vi "main(debug2_chagne_gen3_format).vi"() -> ()   [LabVIEW 2015]
panel:
  out "삭제된 부분":string[][](array[string])
  out "Filtered Sensor":u32[][](array[numeric])
  out "No Filter Sensor":u32[][](array[numeric])
  out "Time":string[](array[string])
  out "배열":string[](array[string])
  in  "패턴(*.txt)":string="*.txt"
  out "파일 이름":string[](array[string])
  in  "경로":path
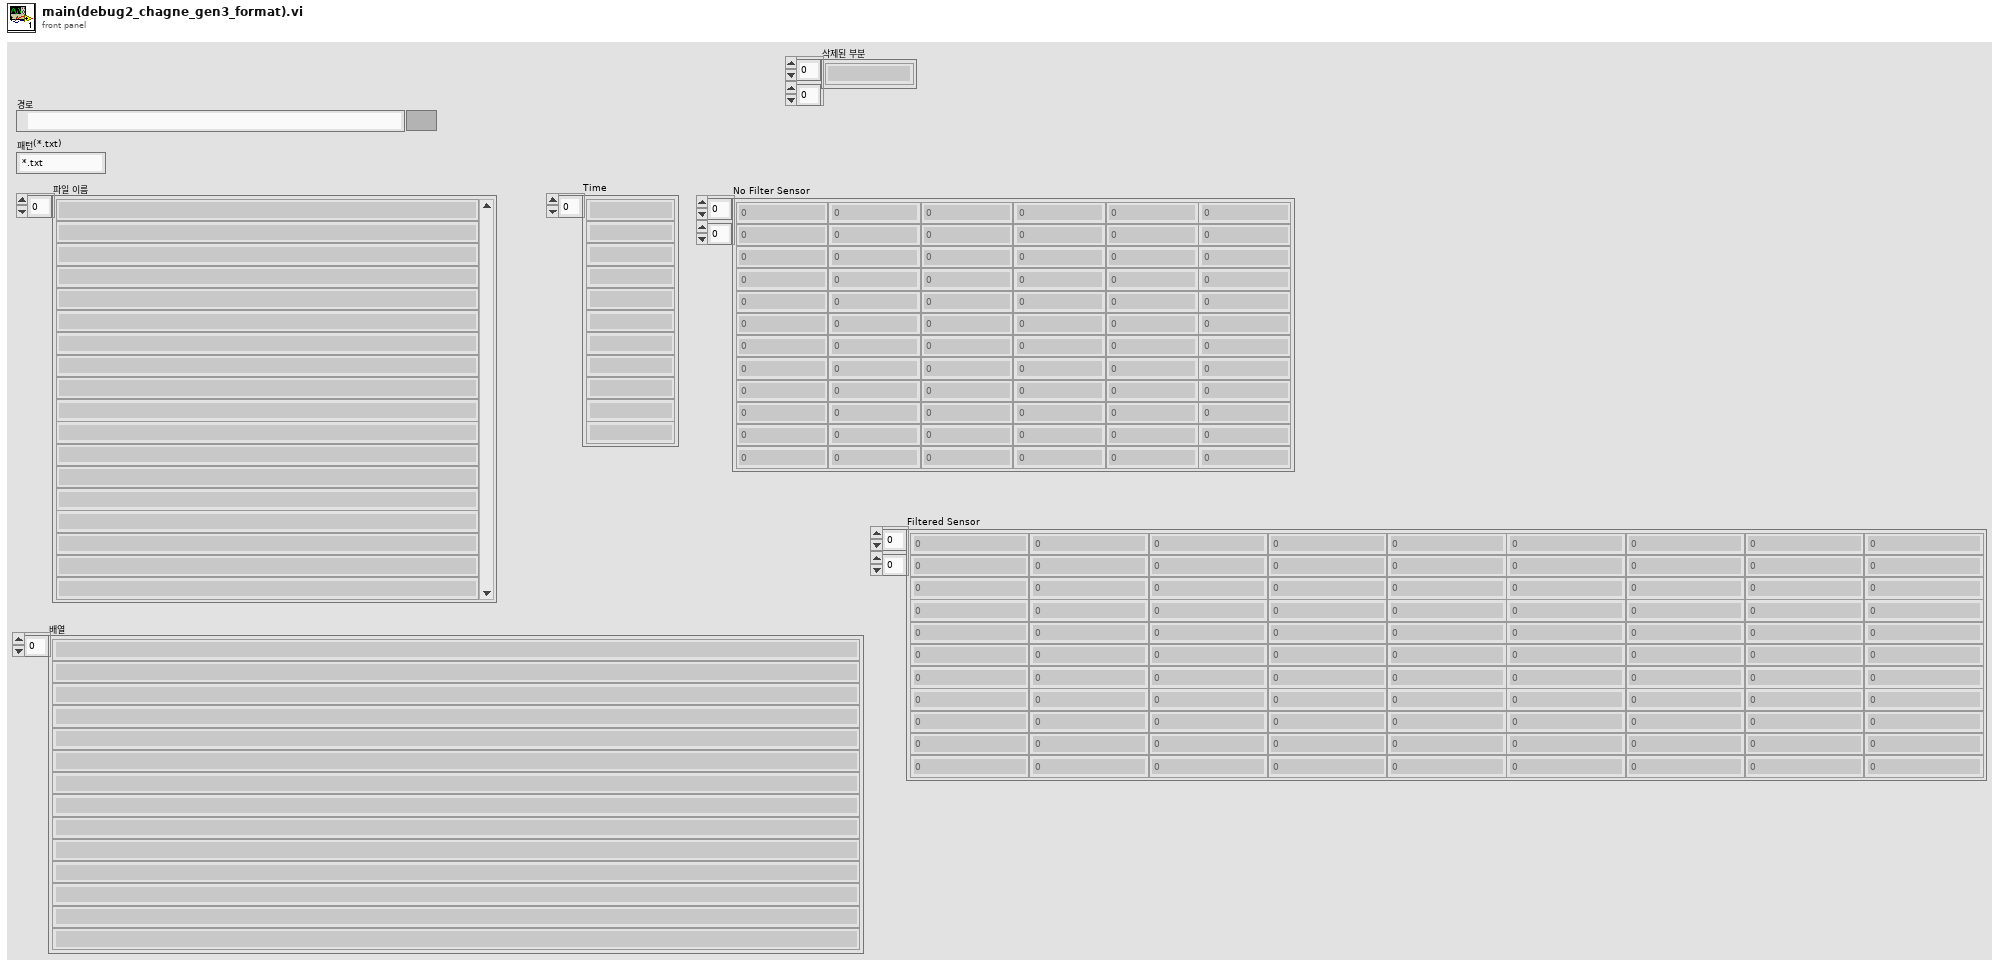
[diagram p1: front panel]
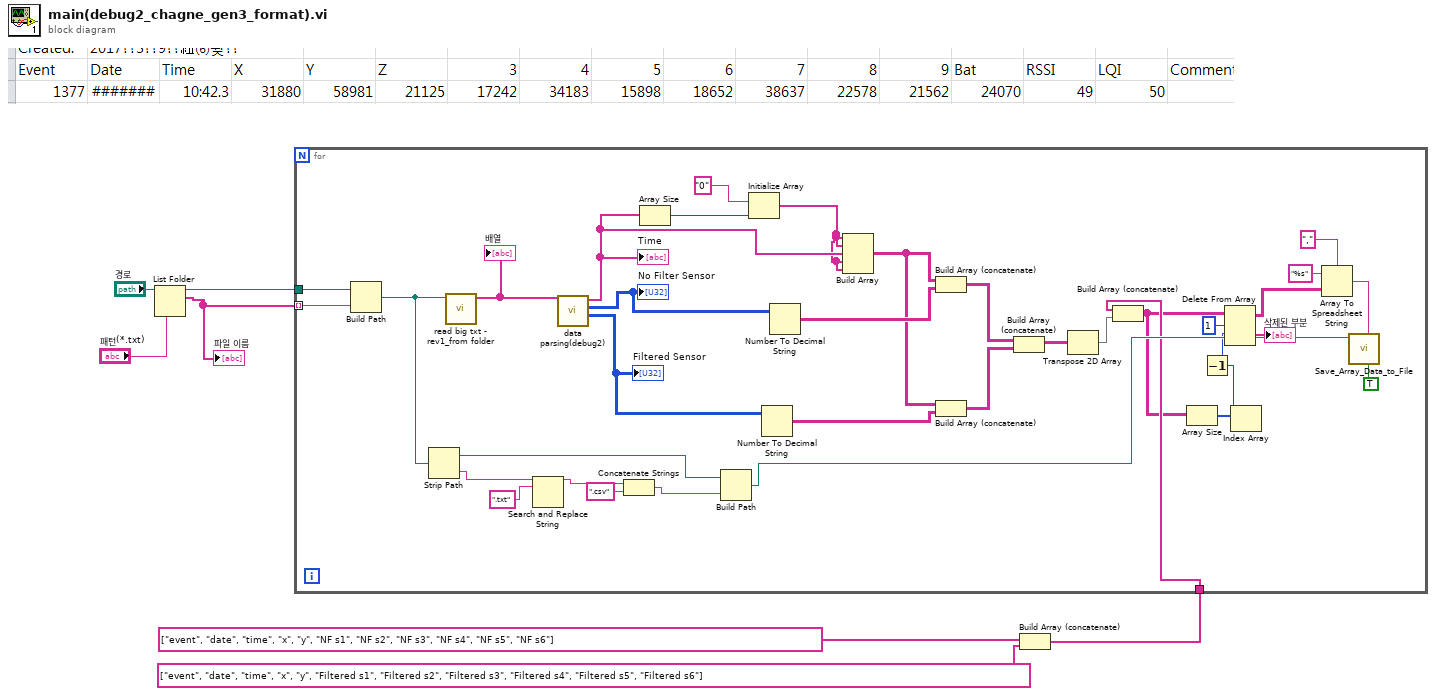
[diagram p0: block diagram]
diagram:
  n1 = List Folder(path="경로", pattern="패턴(*.txt)") -> (path out=w6:path, filenames=w4:string[])  [unwired: 2 in, 2 out]
  "파일 이름" <- w4
  n2 = Build Array (concatenate)(string[] ["event", "date", "time", "x", "y", "NF s1", "NF s2", "NF s3", "NF s4", "NF s5", "NF s6"], string[] ["event", "date", "time", "x", "y", "Filtered s1", "Filtered s2", "Filtered s3", "Filtered s4", "Filtered s5", "Filtered s6"]) -> (w1:string[])
  n3 = for {
    tunnel: w6 -> [w43]
    tunnel: w4 -> [w42] mode=indexing
    tunnel: w1 -> [w15]
    n4 = Build Path(base path=w43, name or relative path=w42) -> (appended path=w28:path)
    n5 = Strip Path(path=w28) -> (stripped path=w23:path, name=w27:string)
    n6 = call "read big txt - rev1_from folder.vi"("파일 경로(대화 상자 사용)"=w28) -> ("배열"=w41:string[])  [unwired: 10 in]
    "배열" <- w41
    n7 = Search and Replace String(input string=w27, search string=".txt" ("검색 문자열")) -> (result string=w25:string)  [unwired: 6 in, 3 out]
    n8 = call "data parsing(debug2).vi"("배열"=w41) -> ("Filtered Sensor"=w35:u32[][], "No Filter Sensor"=w36:u32[][], "Time"=w38:string[])  [unwired: 8 in]
    "Time" <- w38
    "No Filter Sensor" <- w36
    "Filtered Sensor" <- w35
    n9 = Concatenate Strings(w25, ".csv" ("문자열")) -> (w22:string)
    n10 = Array Size(array=w38) -> (size(s)=w40:i32)
    n11 = Build Path(base path=w23, name or relative path=w22) -> (appended path=w21:path)
    n12 = Initialize Array("0", w40) -> (w37:string[])
    n13 = Number To Decimal String(number=w35) -> (decimal integer string=w32:string[][])  [unwired: 1 in]
    n14 = Number To Decimal String(number=w36) -> (decimal integer string=w34:string[][])  [unwired: 1 in]
    n15 = Build Array(w37, w37, w38, w37, w37) -> (w33:string[][])
    n16 = Build Array (concatenate)(w33, w34) -> (w31:string[][])
    n17 = Build Array (concatenate)(w33, w32) -> (w30:string[][])
    n18 = Build Array (concatenate)(w31, w30) -> (w29:string[][])
    n19 = Transpose 2D Array(2D array=w29) -> (transposed array=w16:string[][])
    n20 = Build Array (concatenate)(w15, w16) -> (w13:string[][])
    n21 = Array Size(array=w13) -> (size(s)=w12:i32[])
    n22 = Index Array(array=w12) -> (element=w11:i32)  [unwired: 1 in]
    n23 = Decrement(x=w11) -> (x-1=w10:i32)
    n24 = Delete From Array(array=w13, length=1 ("길이"), index (row)=w10) -> (deleted portion=→"삭제된 부분":string[][], array with subset deleted=w9:string[][])  [unwired: 1 in]
    n25 = Array To Spreadsheet String(delimiter (Tab)="," ("구분 문자(탭)"), array=w9, 3:"%s" ("포맷 문자열")) -> (spreadsheet string=w18:string)
    n26 = call "Save_Array_Data_to_File.vi"("Raw Stiring?"=TRUE, "Raw String"=w18, "file path (use dialog)"=w21) -> ()  [unwired: 8 in, 1 out]
  }
